vi "TDTSyn-Get Events (Client Side).vi"(0 "IP Address":string, 5 "Port":i32, 7 "last read":bool, 11 "error in (no error)":errorcluster) -> (4 "Codes":i16[](array[numeric]), 8 "Times":sgl[](array[numeric]), 15 "error out":errorcluster)   [LabVIEW 2020]
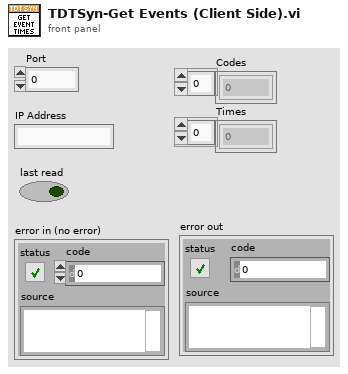
[diagram p1: front panel]
types:
  T1 = enum16{"big-endian, network order", "native, host order", "little-endian"}
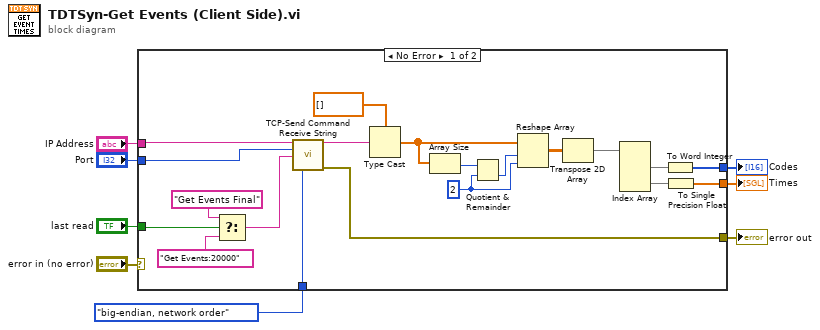
[diagram p0: block diagram]
diagram:
  n1 = case shown="No Error" "error in (no error)" {
    selector: "error in (no error)" -> [_ w29]
    tunnel: "IP Address" -> [w26 _]
    tunnel: "Port" -> [w25 _]
    tunnel: "last read" -> [w28 _]
    tunnel: [w22 w29] -> w4
    tunnel: [w12 _] -> w3
    tunnel: [w11 _] -> w2
    tunnel: T1."big-endian, network order" ("byte order") -> [w9 _]
    frame No Error {
      w17 = 2 ("dimension size")
      n2 = Select(t="Get Events Final" ("Command"), s=w28, f="Get Events:20000" ("Command")) -> (s? t:f=w10:string)
      n3 = call "TCP-Send Command Receive String.vi"("PXI Address"=w26, "Port"=w25, "Command"=w10, "byte order"=w9) -> ("data"=w24:string, "error out"=w22:errorcluster)  [unwired: 10 in]
      n4 = Type Cast(type=dbl[] [], x=w24) -> (*(type *) &x=w16:dbl[])
      n5 = Array Size(array=w16) -> (size(s)=w19:i32)
      n6 = Quotient & Remainder(x=w19, y=w17) -> (floor(x/y)=w18:i32)  [unwired: 1 out]
      n7 = Reshape Array(w16, w18, w17) -> (w20:dbl[][])
      n8 = Transpose 2D Array(2D array=w20) -> (transposed array=w15:dbl[][])
      n9 = Index Array(array=w15) -> (element #1=w14:dbl[], element #2=w13:dbl[])  [unwired: 4 in]
      n10 = To Word Integer(number=w14) -> (16bit integer=w12:i16[])
      n11 = To Single Precision Float(number=w13) -> (single precision float=w11:sgl[])
    }
    frame Error {
    }
  }
  "error out" <- w4
  "Codes" <- w3
  "Times" <- w2
